vi "Create Border Line.vi"(7 "3D Waterfall Property":T4={"General Property"={"Plot Name"="", "Coordinate System"=enum."Cartesian", "Opacity"=0.0}, "Projection Property"={"Draw XY"=FALSE, "Draw YZ"=FALSE, "Draw XZ"=FALSE}, "Plot Property"={"Line Style"=enum."None", "Line Width"=0.0, "Color Ramp Cluster"={"Color Ramp Style"=enum."None", "Color Ramp Array"=[16711934, 393471, 57855, 4390754, 16449346, 16744722, 16711680], "Color Ramp Index"=[45, 91, 133, 175, 219, 255], "Interpolate?"=FALSE, "Logarithm?"=FALSE}, "Antialiasing"=FALSE}, "Waterfall Property"={"Waterfall Mode"=enum."Lines"}}, 8 "error in (no error)":errorcluster, 9 "Actual Transform In":T7, 10 "Plot Representation In":T1, 11 "Plot Object In":refnum<vi>) -> (0 "error out":errorcluster, 1 "Actual Transform Out":T7, 2 "Plot Representation Out":T1, 3 "Plot Object Out":refnum<vi>, 4 "Border Line Object Out":refnum<vi>)   [LabVIEW 2020, in "3D Waterfall.lvclass"]
uses:
  <vilib>/Math Plots/3D Math Plots/3D Waterfall/3D Waterfall/3D Waterfall.lvclass
  <vilib>/Math Plots/3D Math Plots/3D Plot/3D Plot/Typedef/Actual Transform.ctl
  <vilib>/Math Plots/3D Math Plots/3D Plot/3D Plot/Typedef/Range Clusters.ctl
  <vilib>/Math Plots/3D Math Plots/3D Plot/3D Plot/Typedef/Plot Representation.ctl
  <vilib>/Math Plots/3D Math Plots/3D Plot/3D Plot/Typedef/Mesh Data.ctl
  <vilib>/Math Plots/3D Math Plots/3D Waterfall/3D Waterfall/Typedef/3D Waterfall Property.ctl
  <vilib>/Math Plots/3D Math Plots/3D Plot/3D Plot/Typedef/Line Type.ctl
  <vilib>/Math Plots/3D Math Plots/3D Plot/3D Plot/Typedef/Color Ramp Cluster.ctl
  <vilib>/picture/3D Picture Control/NI_3D Picture Control.lvlib
  <vilib>/Math Plots/3D Math Plots/3D Plot/3D Plot/3D Plot.lvclass
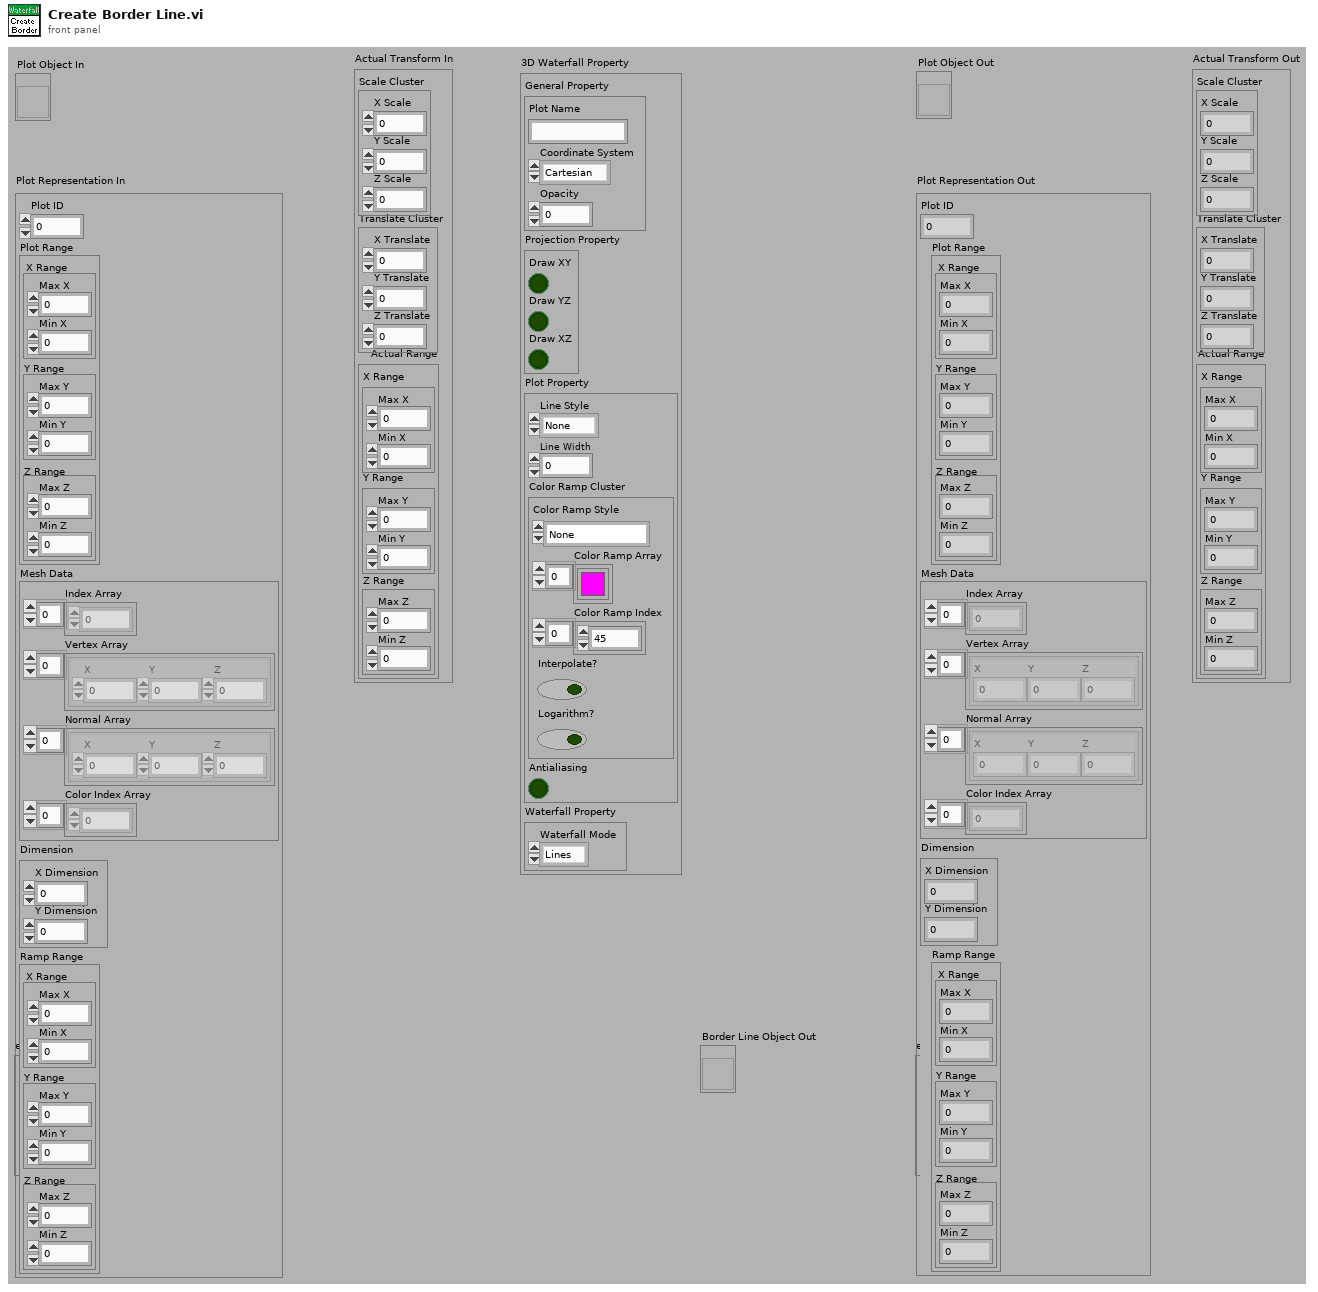
[diagram p1: front panel]
types:
  T1 = typedef "3D Plot.lvclass/Plot Representation.ctl" = cluster{"Plot ID":i32, "Plot Range":T2, "Mesh Data":T3, "Dimension":cluster{"X Dimension":i32, "Y Dimension":i32}, "Ramp Range":T2}
  T2 = typedef "3D Plot.lvclass/Range Clusters.ctl" = cluster{"X Range":cluster{"Max X":sgl, "Min X":sgl}, "Y Range":cluster{"Max Y":sgl, "Min Y":sgl}, "Z Range":cluster{"Max Z":sgl, "Min Z":sgl}}
  T3 = typedef "3D Plot.lvclass/Mesh Data.ctl" = cluster{"Index Array":u32[], "Vertex Array":cluster{"X":sgl, "Y":sgl, "Z":sgl}[], "Normal Array":cluster{"X":sgl, "Y":sgl, "Z":sgl}[], "Color Index Array":i32[]}
  T4 = typedef "3D Waterfall.lvclass/3D Waterfall Property.ctl" = cluster{"General Property":cluster{"Plot Name":string, "Coordinate System":enum16{"Cartesian", "Cylindrical", "Spherical"}, "Opacity":sgl}, "Projection Property":cluster{"Draw XY":bool, "Draw YZ":bool, "Draw XZ":bool}, "Plot Property":cluster{"Line Style":T5, "Line Width":sgl, "Color Ramp Cluster":T6, "Antialiasing":bool}, "Waterfall Property":cluster{"Waterfall Mode":enum16{"Lines", "Slices"}}}
  T5 = typedef "3D Plot.lvclass/Line Type.ctl" = enum16{"None", "Solid", "Dash", "Dot", "Dash Dot"}
  T6 = typedef "3D Plot.lvclass/Color Ramp Cluster.ctl" = cluster{"Color Ramp Style":enum16{"None", "Shaded", "Color spectrum", "Grey scale", "Custom"}, "Color Ramp Array":u32[], "Color Ramp Index":i32[], "Interpolate?":bool, "Logarithm?":bool}
  T7 = typedef "3D Plot.lvclass/Actual Transform.ctl" = cluster{"Scale Cluster":cluster{"X Scale":sgl, "Y Scale":sgl, "Z Scale":sgl}, "Translate Cluster":cluster{"X Translate":sgl, "Y Translate":sgl, "Z Translate":sgl}, "Actual Range":T2}
  T8 = enum16{"Overall", "Per Primitive", "Per Vertex", "Binding Off"}
  T9 = enum16{"Points", "Lines", "Line Strip", "Line Loop", "Triangles", "Triangle Strip", "Triangle Fan", "Quads", "Quad Strip", "Polygon"}
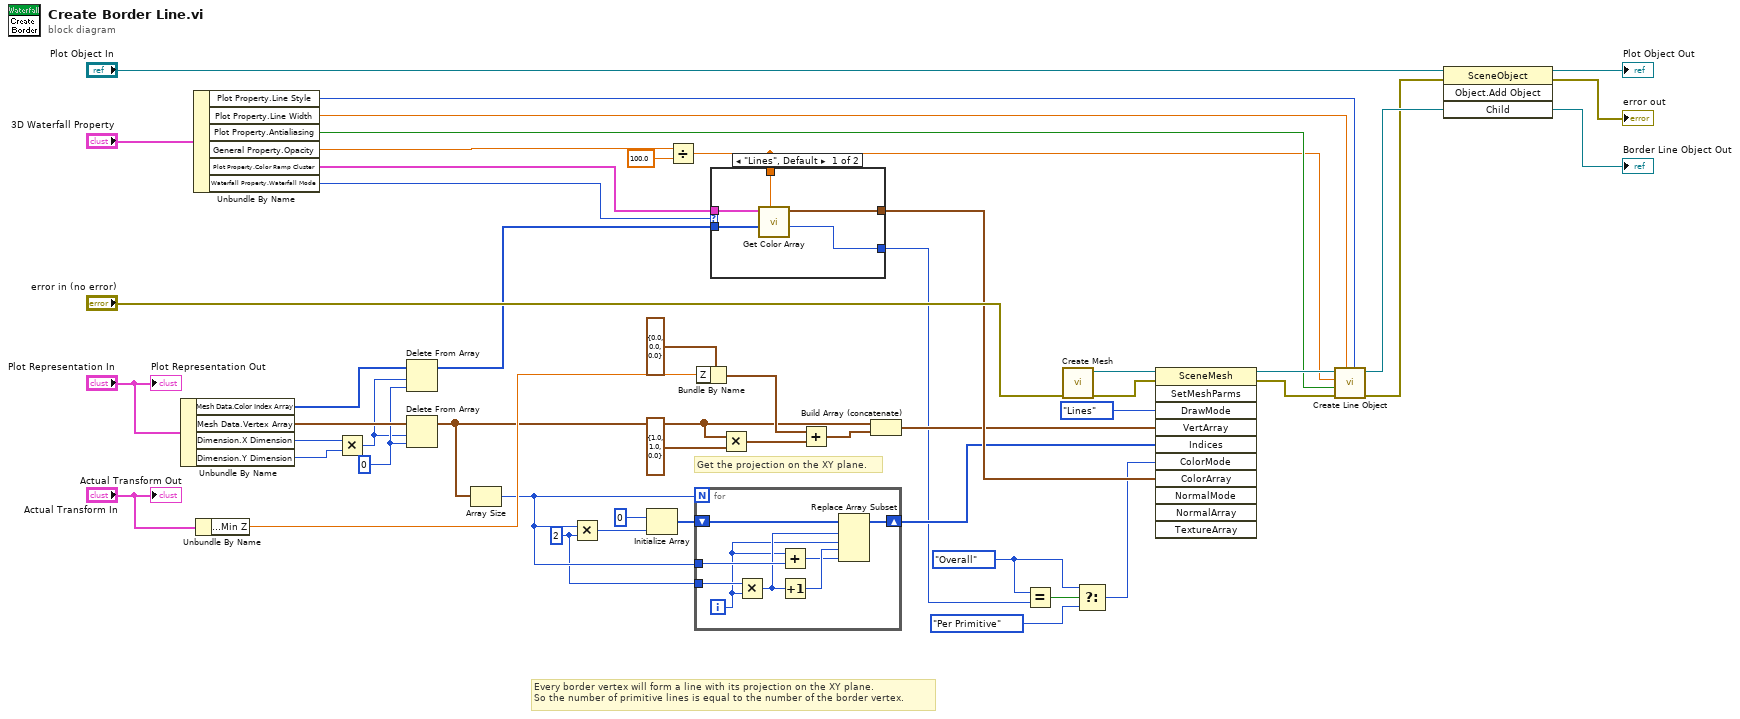
[diagram p0: block diagram]
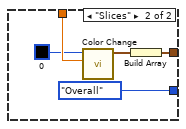
[diagram p2: hidden frame]
diagram:
  w4 = 0 ("index")
  w10 = 2 ("y")
  w21 = T8."Overall" ("y")
  # "Get the projection on the XY plane."
  # "Every border vertex will form a line with its projection on the XY plane. \nSo the number of primitive lines is equal to the number of the border vertex."
  n1 = Unbundle By Name("Plot Representation In") -> ("Mesh Data.Color Index Array"=w6:i32[], "Mesh Data.Vertex Array"=w5:cluster{"X":sgl, "Y":sgl, "Z":sgl}[], "Dimension.X Dimension"=w41:i32, "Dimension.Y Dimension"=w8:i32)
  n2 = Unbundle By Name("3D Waterfall Property") -> ("Plot Property.Line Style"=w25:T5, "Plot Property.Line Width"=w26:sgl, "Plot Property.Antialiasing"=w18:bool, "General Property.Opacity"=w24:sgl, "Plot Property.Color Ramp Cluster"=w9:T6, "Waterfall Property.Waterfall Mode"=w7:enum16{"Lines", "Slices"})
  n3 = Unbundle By Name("Actual Transform In") -> ("Actual Range.Z Range.Min Z"=w33:sgl)
  n4 = Multiply(x=w41, y=w8) -> (x*y=w3:i32)
  n5 = Delete From Array(array=w6, length=w3, index=w4) -> (array with subset deleted=w2:i32[])  [unwired: 1 out]
  n6 = Delete From Array(array=w5, length=w3, index=w4) -> (array with subset deleted=w1:cluster{"X":sgl, "Y":sgl, "Z":sgl}[])  [unwired: 1 out]
  n7 = Array Size(array=w1) -> (size(s)=w13:i32)
  n8 = Multiply(x=w13, y=w10) -> (x*y=w12:i32)
  n9 = Initialize Array(u32 0 ("element"), w12) -> (w11:u32[])
  n10 = Divide(x=w24, y=sgl 100.0) -> (x/y=w17:sgl)
  n11 = for {
    N: w13 -> [_]
    shift-right: [w57] -> w34
    shift-left: w11 -> [w58]
    tunnel: w13 -> [w56]
    tunnel: w10 -> [w55]
    i -> [w51]
    n12 = Multiply(x=w55, y=w51) -> (x*y=w54:i32)
    n13 = Add(x=w51, y=w56) -> (x+y=w52:i32)
    n14 = Increment(x=w54) -> (x+1=w53:i32)
    n15 = Replace Array Subset(array=w58, new element #1=w51, index #1=w54, new element #2=w52, index #2=w53) -> (w57:u32[])
  }
  n16 = Bundle By Name(cluster=cluster{"X":sgl, "Y":sgl, "Z":sgl} {"X"=0.0, "Y"=0.0, "Z"=0.0} ("3D Point 2"), "Z"=w33) -> (w36:cluster{"X":sgl, "Y":sgl, "Z":sgl})
  n17 = case shown="\"Lines\", Default" w7 {
    tunnel: [w63 w68] -> w39
    tunnel: w2 -> [w62 _]
    tunnel: [w61 T8."Overall" ("Color Binding Mode")] -> w20
    tunnel: w17 -> [w60 w65]
    tunnel: w9 -> [w59 _]
    frame "Lines", Default {
      n18 = call <vilib>:"Get Color Array.vi"("Alpha"=w60, "Color Index Array"=w62, "Color Ramp Cluster"=w59) -> ("Color Binding Mode"=w61:T8, "Color Array"=w63:cluster{"R":sgl, "G":sgl, "B":sgl, "A":sgl}[])  [unwired: 5 in, 2 out]
    }
    frame "Slices" {
      n19 = call <vilib>:"Color Change.vi"("Alpha"=w65, "Color"=u32 0) -> ("RGBA"=w67:cluster{"R":sgl, "G":sgl, "B":sgl, "A":sgl})  [unwired: 9 out]
      n20 = Build Array(w67) -> (w68:cluster{"R":sgl, "G":sgl, "B":sgl, "A":sgl}[])
    }
  }
  n21 = Multiply(x=w1, y=cluster{"X":sgl, "Y":sgl, "Z":sgl} {"X"=1.0, "Y"=1.0, "Z"=0.0} ("3D Point 2")) -> (x*y=w35:cluster{"X":sgl, "Y":sgl, "Z":sgl}[])
  n22 = Add(x=w36, y=w35) -> (x+y=w37:cluster{"X":sgl, "Y":sgl, "Z":sgl}[])
  n23 = Build Array (concatenate)(w1, w37) -> (w32:cluster{"X":sgl, "Y":sgl, "Z":sgl}[])
  n24 = Equal?(x=w21, y=w20) -> (x = y?=w23:bool)
  n25 = call <vilib>:"Create Mesh.vi"("error in (no error)"="error in (no error)") -> ("error out"=w42:errorcluster, "New Mesh Refnum"=w43:refnum<vi>)  [unwired: 9 out]
  n26 = Select(t=w21, s=w23, f=T8."Per Primitive" ("Color Binding Mode")) -> (s? t:f=w19:T8)
  n27 = invoke class="SceneMesh" method="SetMeshParms"(reference=w43, error in=w42, "DrawMode"=T9."Lines" ("Draw Mode"), "VertArray"=w32, "Indices"=w34, "ColorMode"=w19, "ColorArray"=w39) -> (reference out=w29:refnum<vi>, error out=w30:errorcluster)  [unwired: 4 in, 9 out]
  n28 = call <vilib>:"Create Line Object.vi"("Line Style"=w25, "Line Width"=w26, "error in (no error)"=w30, "Antialiasing"=w18, "Alpha"=w17, "Mesh Ref In"=w29) -> ("error out"=w27:errorcluster, "Object Ref Out"=w28:refnum<vi>)  [unwired: 4 out]
  n29 = invoke class="SceneObject" method="Object.Add Object"(reference="Plot Object In", error in=w27, "Child"=w28) -> (reference out=→"Plot Object Out":refnum<vi>, error out=→"error out":errorcluster, "Child"=→"Border Line Object Out":refnum<vi>)  [unwired: 1 in, 1 out]
  "Actual Transform Out" <- "Actual Transform In"
  "Plot Representation Out" <- "Plot Representation In"
